vi "获取引用簇.vi"(8 "错误输入（无错误）":errorcluster, 10 "文件路径":path, 11 "Excel._Application":refnum<k7>) -> (0 "错误输出":errorcluster, 3 "引用簇":T1)   [LabVIEW 2021, in "OperateExcel.lvlib"]
uses:
  OperateExcel.lvlib
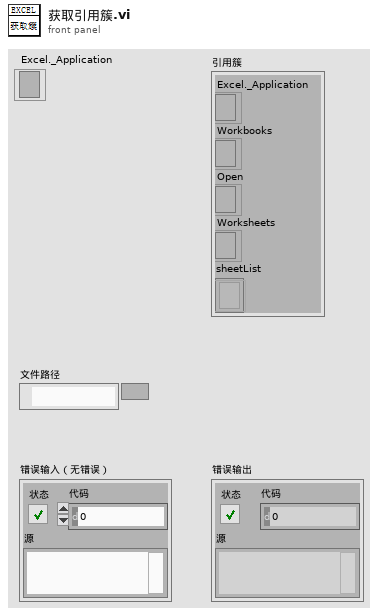
[diagram p1: front panel]
types:
  T1 = typedef "OperateExcel.lvlib/引用簇.ctl" = cluster{"Excel._Application":refnum<k7>, "Workbooks":refnum<k7>, "Open":refnum<k7>, "Worksheets":refnum<k7>, "sheetList":refnum<k7>[]}
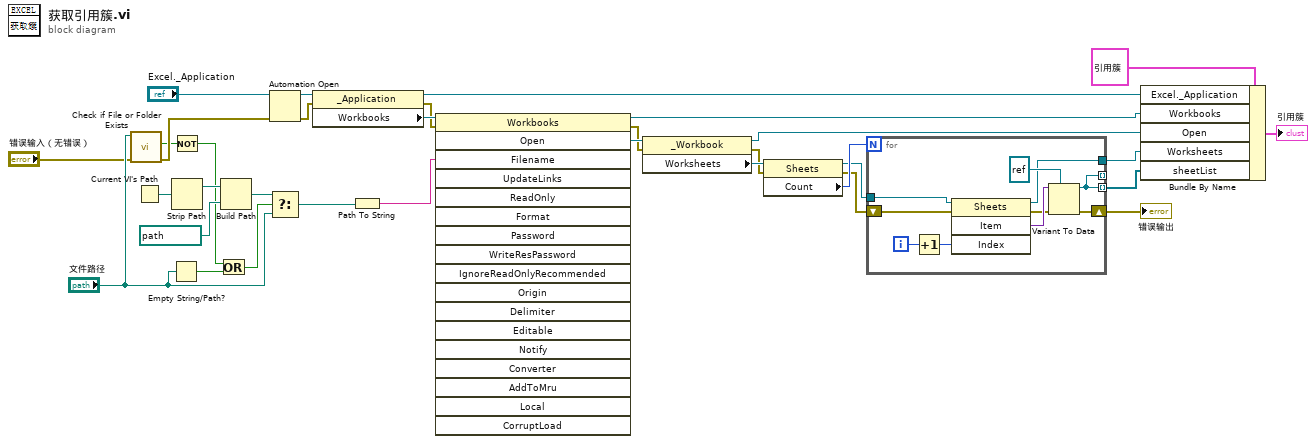
[diagram p0: block diagram]
diagram:
  n1 = call <vilib>:"Check if File or Folder Exists.vi"("error in (no error)"="错误输入（无错误）", "path"="文件路径") -> ("error out"=w9:errorcluster, "file or folder exists?"=w2:bool)  [unwired: 7 in, 1 out]
  n2 = Current VI's Path() -> (path=w4:path)
  n3 = Empty String/Path?(string/path="文件路径") -> (empty?=w8:bool)
  n4 = Not(x=w2) -> (.not. x?=w1:bool)
  n5 = Strip Path(path=w4) -> (stripped path=w3:path)  [unwired: 1 out]
  n6 = Or(x=w1, y=w8) -> (x .or. y?=w7:bool)
  n7 = Build Path(base path=w3, name or relative path=path "模板.xlsx" ("文件路径")) -> (appended path=w5:path)
  n8 = Automation Open(error in (no error)=w9, Automation Refnum="Excel._Application") -> (Automation Refnum=w15:refnum<k7>, error out=w14:errorcluster)  [unwired: 2 in]
  n9 = Select(t=w5, s=w7, f="文件路径") -> (s? t:f=w12:path)
  n10 = property class="_Application"(reference=w15, error in=w14) -> (reference out=w22:refnum<k7>, error out=w30:errorcluster, "Workbooks"=w33:refnum<k7>)
  n11 = Path To String(path=w12) -> (string=w32:string)
  n12 = invoke class="Workbooks" method="Open"(reference=w33, error in=w30, "Filename"=w32) -> (reference out=w21:refnum<k7>, error out=w29:errorcluster, "Open"=w31:refnum<k7>)  [unwired: 15 in, 15 out]
  n13 = property class="_Workbook"(reference=w31, error in=w29) -> (reference out=w20:refnum<k7>, error out=w27:errorcluster, "Worksheets"=w28:refnum<k7>)
  n14 = property class="Sheets"(reference=w28, error in=w27) -> (reference out=w25:refnum<k7>, error out=w24:errorcluster, "Count"=w26:i32)
  n15 = for {
    N: w26 -> [_]
    tunnel: w25 -> [w43]
    tunnel: [w34] -> _ mode=indexing
    shift-right: [w36] -> w23
    shift-left: w24 -> [w42]
    tunnel: [w35] -> w19
    tunnel: [w34] -> w18 mode=indexing
    i -> [w41]
    n16 = Increment(x=w41) -> (x+1=w40:i32)
    n17 = invoke class="Sheets" method="Item"(reference=w43, error in=w42, "Index"=w40) -> (reference out=w35:refnum<k7>, error out=w37:errorcluster, "Item"=w39:variant)  [unwired: 1 in, 1 out]
    n18 = Variant To Data(error in=w37, type=refnum<k7> refnum ("引用输出"), Variant=w39) -> (data=w34:refnum<k7>, error out=w36:errorcluster)
  }
  "错误输出" <- w23
  n19 = Bundle By Name(cluster=T1 {"Excel._Application"=refnum, "Workbooks"=refnum, "Open"=refnum, "Worksheets"=refnum, "sheetList"=[refnum]} ("引用簇"), "Excel._Application"=w22, "Workbooks"=w21, "Open"=w20, "Worksheets"=w19, "sheetList"=w18) -> (→"引用簇":T1)
